vi "BRig_Host__Loop_Consumer_RunState__closedLoop_getInputTrialList.vi"(8 "input_nTrial":u16, 10 "input_trialList":u16[](array[numeric]), 11 "input_updateID":u16) -> (0 "output_trialList":string, 2 "output_trialList":u16[](array[numeric]), 3 "output_updateID":u16)   [LabVIEW 2014]
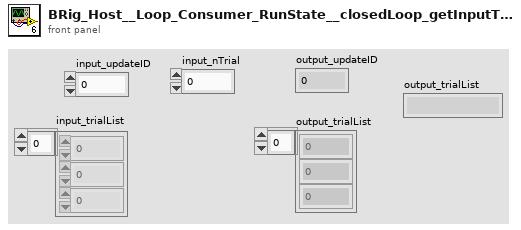
[diagram p1: front panel]
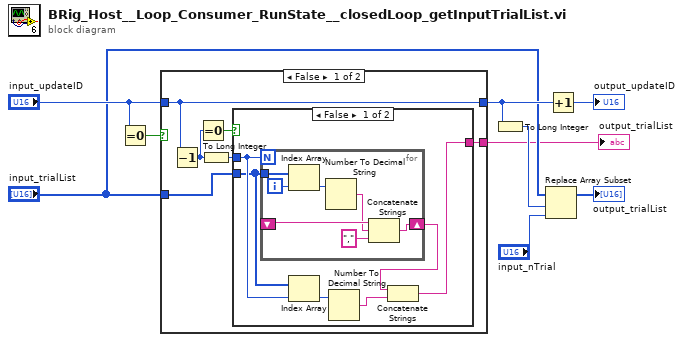
[diagram p0: block diagram]
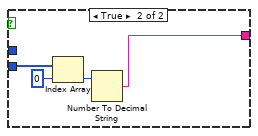
[diagram p2: hidden frame]
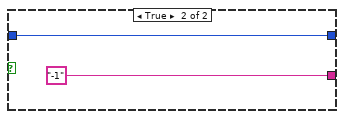
[diagram p3: hidden frame]
diagram:
  n1 = Equal To 0?(x="input_updateID") -> (x = 0?=w9:bool)
  n2 = case shown="False" w9 {
    tunnel: [w10 "-1"] -> w1
    tunnel: "input_trialList" -> [w11 _]
    tunnel: "input_updateID" -> [w15 w33]
    tunnel: [w15 w33] -> w7
    frame False {
      n3 = Decrement(x=w15) -> (x-1=w13:u16)
      n4 = Equal To 0?(x=w13) -> (x = 0?=w14:bool)
      n5 = To Long Integer(number=w13) -> (32bit integer=w12:i32)
      n6 = case shown="False" w14 {
        tunnel: w12 -> [w21 _]
        tunnel: w11 -> [w20 w32]
        tunnel: [w16 w29] -> w10
        frame False {
          n7 = for {
            N: w21 -> [_]
            tunnel: w20 -> [w28]
            shift-right: [w23] -> w17
            shift-left: _ -> [w25]
            i -> [w27]
            n8 = Index Array(array=w28, index=w27) -> (element=w26:u16)
            n9 = Number To Decimal String(number=w26) -> (decimal integer string=w24:string)  [unwired: 1 in]
            n10 = Concatenate Strings(w25, w24, "," ("string")) -> (w23:string)
          }
          n11 = Index Array(array=w20, index=w21) -> (element=w19:u16)
          n12 = Number To Decimal String(number=w19) -> (decimal integer string=w18:string)  [unwired: 1 in]
          n13 = Concatenate Strings(w17, w18) -> (w16:string)
        }
        frame True {
          n14 = Index Array(array=w32, index=0) -> (element=w30:u16)
          n15 = Number To Decimal String(number=w30) -> (decimal integer string=w29:string)  [unwired: 1 in]
        }
      }
    }
    frame True {
    }
  }
  "output_trialList" <- w1
  n16 = To Long Integer(number=w7) -> (32bit integer=w6:i32)
  n17 = Replace Array Subset(array="input_trialList", new element="input_nTrial", index=w6) -> (→"output_trialList":u16[])
  n18 = Increment(x=w7) -> (x+1=→"output_updateID":u16)
